vi "TP_Calibration.vi"(9 "PEU":refnum<class "PEU.lvclass">, 10 "TP":string, 11 "E5071C":refnum<class "E5071C.lvclass">) -> (3 "Calibration Done":bool)   [LabVIEW 2020]
uses:
  Driver/E5071C/E5071C/E5071C.lvclass
  Driver/PEU/PEU/PEU.lvclass
panel:
  in  "返回":bool
  in  "THROUGH":bool
  in  "LOAD 2":bool
  in  "SHORT 2":bool
  in  "LOAD 1":bool
  in  "SHORT 1":bool
  in  "OPEN 2":bool
  out "TP1":string
  out "TP2":string
  in  "OPEN 1":bool
  in  "确认":bool
  # "E5071C校准"
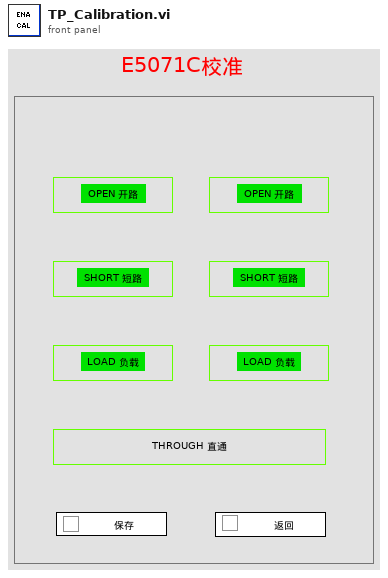
[diagram p1: front panel]
types:
  T1 = enum8{"Enabled", "Disabled", "Disabled and Grayed Out"}
  T2 = cluster{"E5071C":refnum<class "E5071C.lvclass">, "Button Name":string, ":SENS":i32, "Calibration Done":bool, "Done Count":string[]}
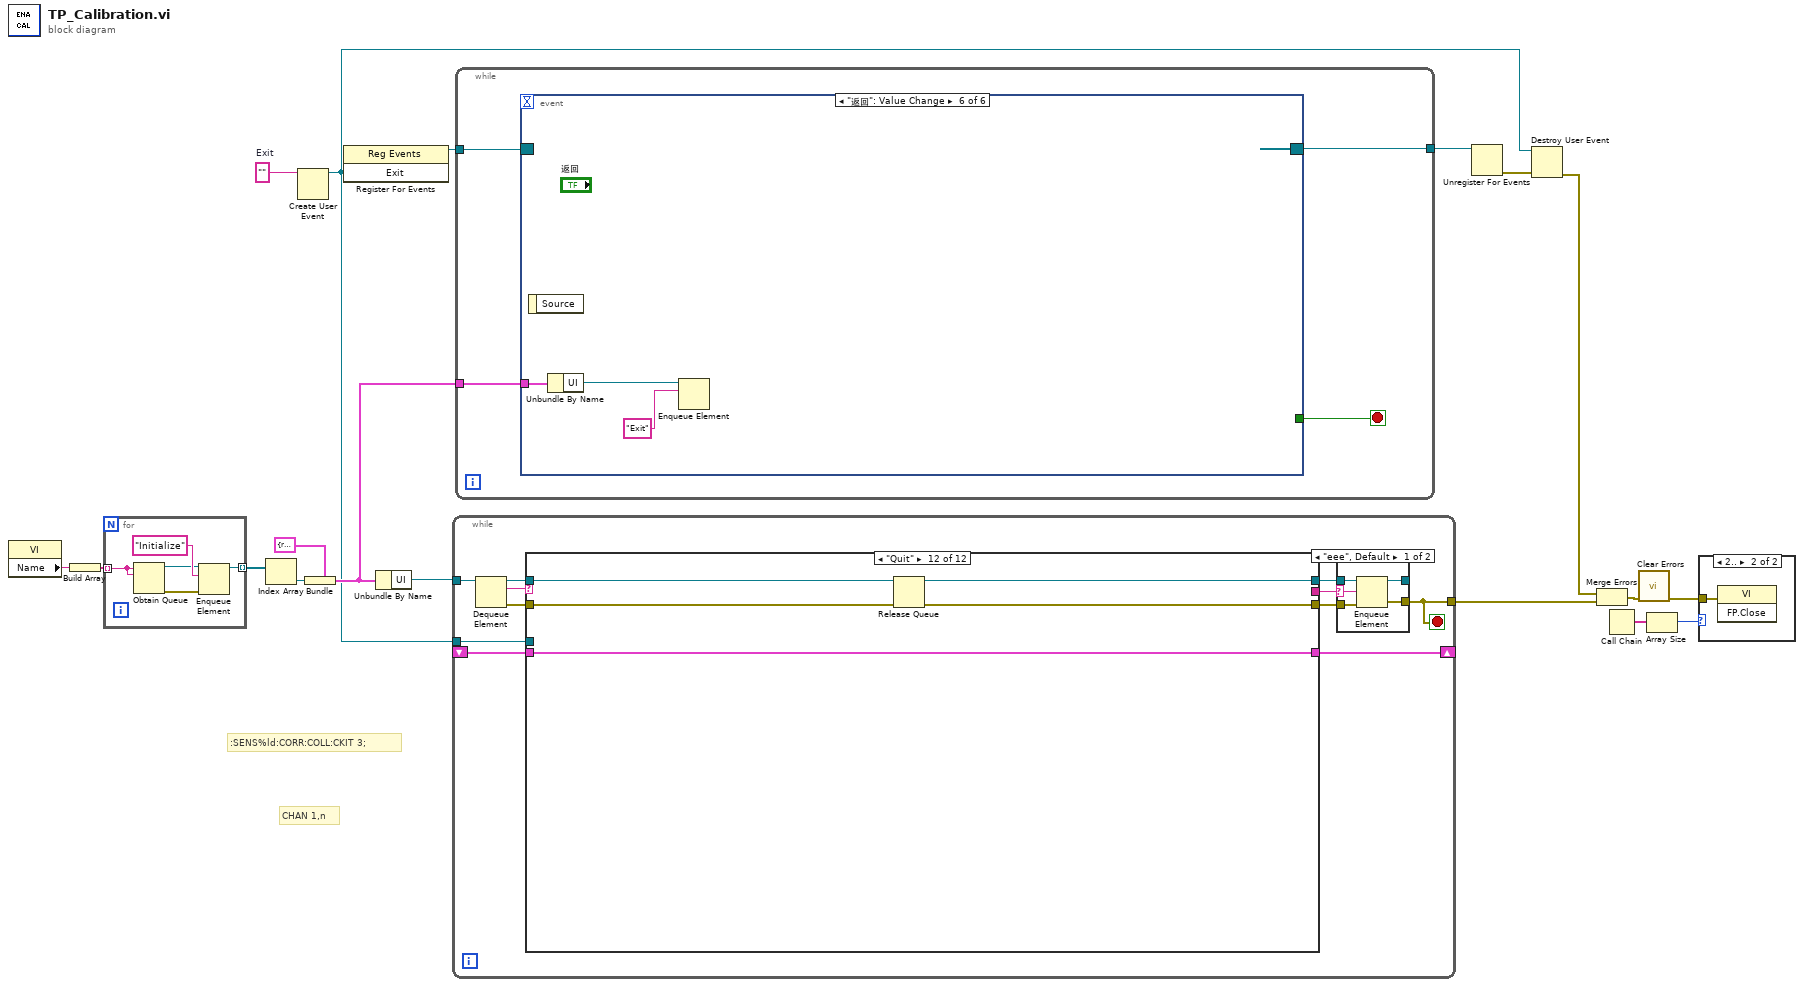
[diagram p0: block diagram]
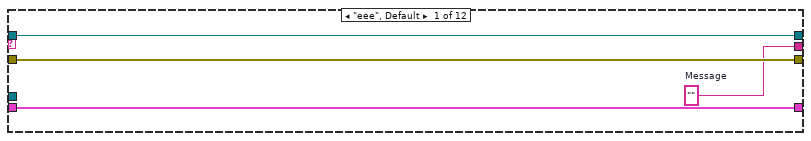
[diagram p4: hidden frame]
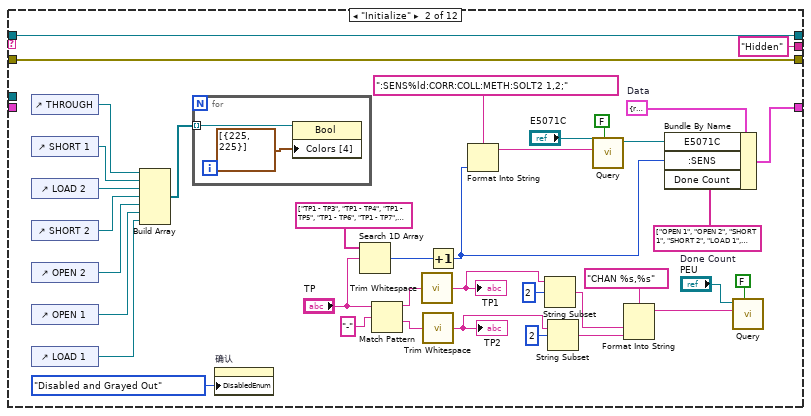
[diagram p5: hidden frame]
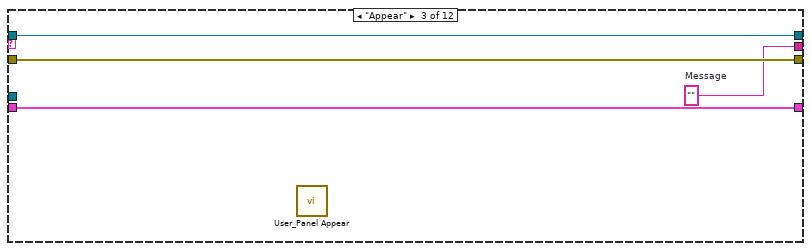
[diagram p6: hidden frame]
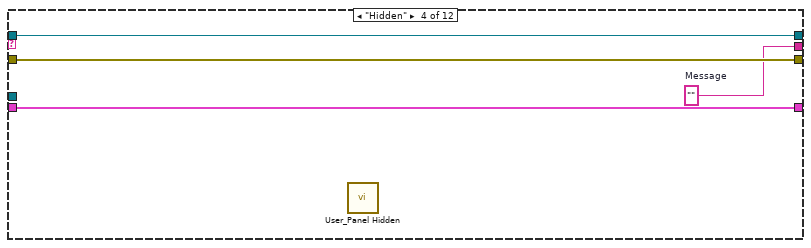
[diagram p7: hidden frame]
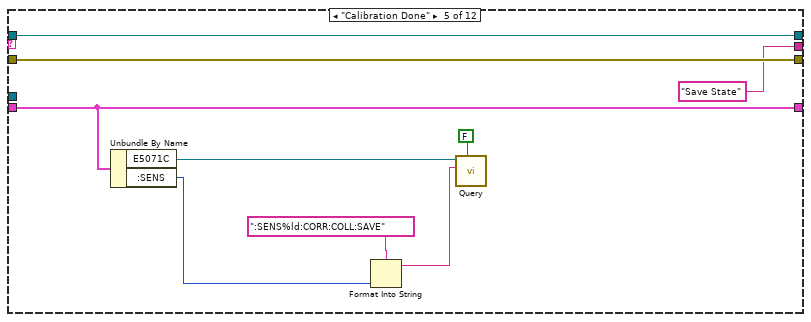
[diagram p8: hidden frame]
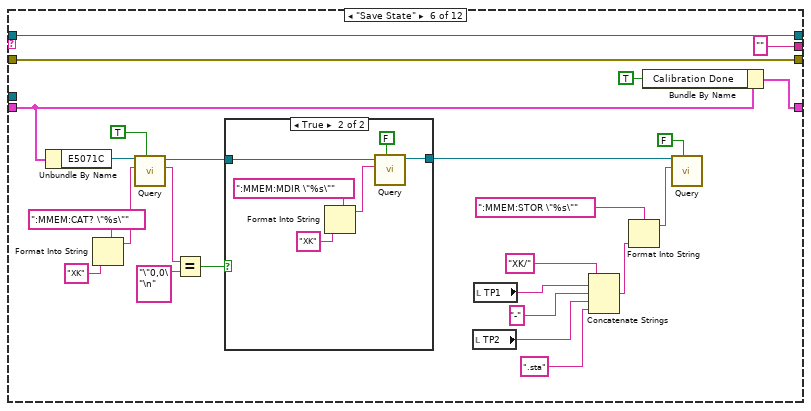
[diagram p9: hidden frame]
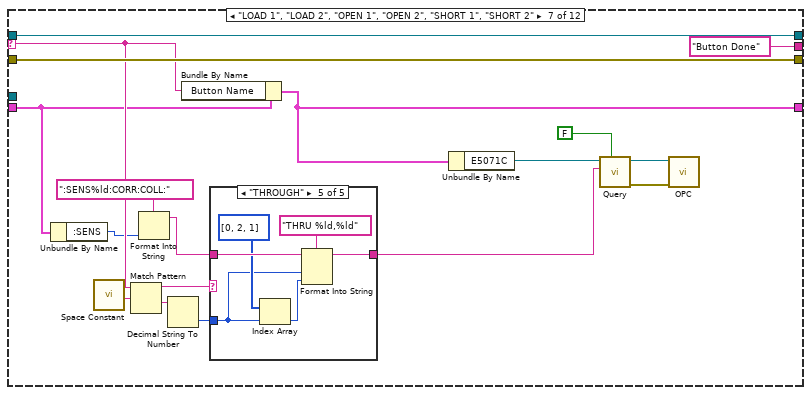
[diagram p11: hidden frame]
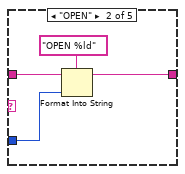
[diagram p13: hidden frame]
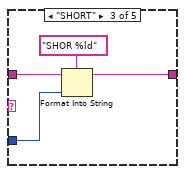
[diagram p14: hidden frame]
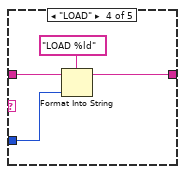
[diagram p15: hidden frame]
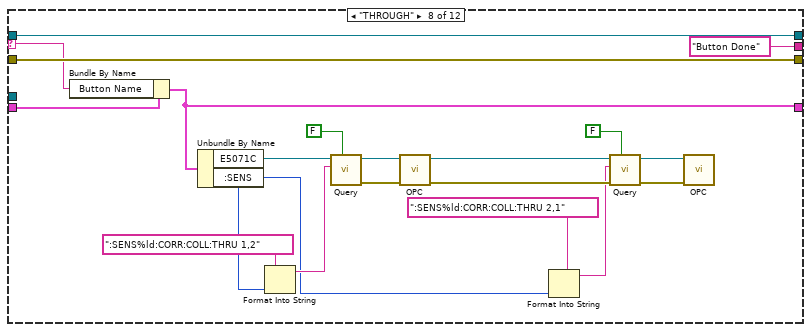
[diagram p16: hidden frame]
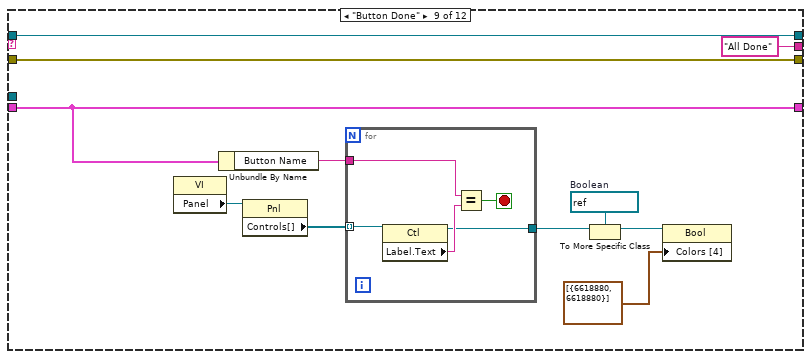
[diagram p17: hidden frame]
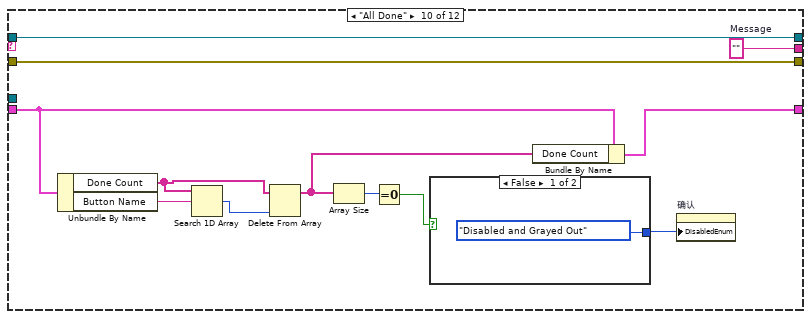
[diagram p18: hidden frame]
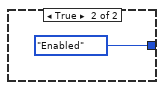
[diagram p19: hidden frame]
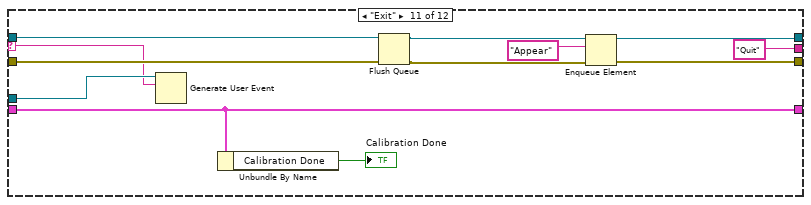
[diagram p20: hidden frame]
diagram:
  w7 = ""  # Exit
  # "CHAN 1,n"
  # ":SENS%ld:CORR:COLL:CKIT 3;"
  n1 = property class="VI"() -> ("Name"=w17:string)  [unwired: 2 in, 2 out]
  n2 = Build Array(w17) -> (w18:string[])
  n3 = for {
    tunnel: w18 -> [w19] mode=indexing
    tunnel: [w20] -> w12 mode=indexing
    n4 = Obtain Queue(name (unnamed)=w19, element data type=w19) -> (queue out=w22:refnum<queue>, error out=w21:errorcluster)  [unwired: 3 in, 1 out]
    n5 = Enqueue Element(queue=w22, element="Initialize" ("元素"), error in (no error)=w21) -> (queue out=w20:refnum<queue>)  [unwired: 1 in, 2 out]
  }
  n6 = Index Array(array=w12) -> (element=w15:refnum<queue>)  [unwired: 1 in]
  n7 = Create User Event(user event datatype=w7) -> (user event=w11:refnum<user-event>)  [unwired: 1 in, 1 out]
  n8 = Bundle(cluster=cluster{"UI":refnum<queue>} {"UI"=refnum}, "UI"=w15) -> (w16:cluster{"UI":refnum<queue>})
  n9 = register-events(w11) -> (reference out=w8:refnum<event-registration>)  [unwired: 2 in, 1 out]
  n10 = Unbundle By Name(w16) -> ("UI"=w13:refnum<queue>)
  n11 = while {
    tunnel: w13 -> [w34]
    tunnel: [w24] -> w1
    shift-right: [w28] -> _
    shift-left: _ -> [w27]
    tunnel: w11 -> [w26]
    stop <- w24 stop-if-true
    n12 = Dequeue Element(queue=w34) -> (queue out=w33:refnum<queue>, element=w25:string, error out=w30:errorcluster)  [unwired: 2 in, 1 out]
    n13 = case shown="\"Quit\"" w25 {
      selector: w25 -> [_ _ _ _ _ _ w142 w184 _ _ w227 _]
      tunnel: w33 -> [w45 w82 w88 w92 w101 w126 w151 w189 w200 w217 w230 w235]
      tunnel: [w45 w82 w88 w92 w101 w126 w151 w189 w200 w217 w222 w235] -> w32
      tunnel: [w44 w81 w87 w91 w100 w125 w150 w188 w199 w216 w224 w232] -> w31
      tunnel: w30 -> [w44 w81 w87 w91 w100 w125 w150 w188 w199 w216 w229 w234]
      tunnel: [w43 "Hidden" ("Message") w86 w90 "Save State" ("Message") "" ("Message") "Button Done" ("Message") "Button Done" ("Message") "All Done" ("Message") w215 "Quit" ("Message") _] -> w29
      tunnel: [w42 w78 w85 w89 w98 w103 w141 w183 w197 w211 w221 w233] -> w28
      tunnel: w27 -> [w42 _ w85 w89 w98 w104 w137 w185 w197 w212 w221 w233]
      tunnel: w26 -> [_ _ _ _ _ _ _ _ _ _ w228 _]
      frame "eee", Default {
        w43 = ""  # Message
      }
      frame "Initialize" {
        w65 = string[] ["OPEN 1", "OPEN 2", "SHORT 1", "SHORT 2", "LOAD 1", "LOAD 2", "THROUGH"]  # Done Count
        w79 = T2 {"E5071C"=refnum, "Button Name"="", ":SENS"=0, "Calibration Done"=FALSE, "Done Count"=["OPEN 1", "OPEN 2", "SHORT 1", "SHORT 2", "LOAD 1", "LOAD 2", "THROUGH"]}  # Data
        n14 = control-ref of="THROUGH"() -> (w63:refnum<vi>)
        n15 = control-ref of="SHORT 1"() -> (w62:refnum<vi>)
        n16 = control-ref of="LOAD 2"() -> (w61:refnum<vi>)
        n17 = control-ref of="SHORT 2"() -> (w60:refnum<vi>)
        n18 = control-ref of="OPEN 2"() -> (w59:refnum<vi>)
        n19 = control-ref of="OPEN 1"() -> (w58:refnum<vi>)
        n20 = control-ref of="LOAD 1"() -> (w57:refnum<vi>)
        n21 = Build Array(w63, w62, w61, w60, w59, w58, w57) -> (w56:refnum<vi>[])
        n22 = for {
          tunnel: w56 -> [w84] mode=indexing
          n23 = property class="Bool"(reference=w84, "Colors [4]"=cluster{u32, u32}[] [{225, 225}]) -> ()  [unwired: 1 in, 2 out]
        }
        n24 = property on="确认" class="Bool"("DisabledEnum"=T1."Disabled and Grayed Out" ("Disabled")) -> ()  [unwired: 2 in, 2 out]
        n25 = Search 1D Array(1D array=string[] ["TP1 - TP3", "TP1 - TP4", "TP1 - TP5", "TP1 - TP6", "TP1 - TP7", "TP1 - TP8", "TP1 - TP9", "TP1 - TP10", "TP1 - TP11", "TP1 - TP12", "TP1 - TP13", "TP1 - TP14", "TP2 - TP3", "TP2 - TP4"], element="TP") -> (index of element=w67:i32)  [unwired: 1 in]
        n26 = Match Pattern(string="TP", regular expression="-") -> (before substring=w76:string, after substring=w75:string)  [unwired: 1 in, 2 out]
        n27 = call <vilib>:"Trim Whitespace.vi"("string"=w76) -> ("trimmed string"=w54:string)  [unwired: 1 in]
        "TP1" <- w54
        n28 = call <vilib>:"Trim Whitespace.vi"("string"=w75) -> ("trimmed string"=w52:string)  [unwired: 1 in]
        "TP2" <- w52
        n29 = Increment(x=w67) -> (x+1=w64:i32)
        n30 = Format Into String(format string=":SENS%ld:CORR:COLL:METH:SOLT2 1,2;", w64) -> (resulting string=w73:string)  [unwired: 2 in, 1 out]
        n31 = String Subset(string=w54, offset (0)=2) -> (substring=w48:string)  [unwired: 1 in]
        n32 = String Subset(string=w52, offset (0)=2) -> (substring=w47:string)  [unwired: 1 in]
        n33 = call "Query.vi"("Return"=FALSE, "Command"=w73, "E5071C in"="E5071C") -> ("E5071C out"=w72:refnum<class "E5071C.lvclass">)  [unwired: 6 in, 2 out]
        n34 = Format Into String(format string="CHAN %s,%s", w48, w47) -> (resulting string=w46:string)  [unwired: 2 in, 1 out]
        n35 = Bundle By Name(cluster=w79, "E5071C"=w72, ":SENS"=w64, "Done Count"=w65) -> (w78:T2)
        n36 = call "Query.vi"("Return"=FALSE, "Command"=w46, "PEU in"="PEU") -> ()  [unwired: 6 in, 3 out]
      }
      frame "Appear" {
        w86 = ""  # Message
        n37 = call "User_Panel Appear.vi"() -> ()  [unwired: 11 in, 1 out]
      }
      frame "Hidden" {
        w90 = ""  # Message
        n38 = call "User_Panel Hidden.vi"() -> ()  [unwired: 11 in, 1 out]
      }
      frame "Calibration Done" {
        n39 = Unbundle By Name(w98) -> ("E5071C"=w97:refnum<class "E5071C.lvclass">, ":SENS"=w94:i32)
        n40 = Format Into String(format string=":SENS%ld:CORR:COLL:SAVE" ("element"), w94) -> (resulting string=w93:string)  [unwired: 2 in, 1 out]
        n41 = call "Query.vi"("Return"=FALSE, "Command"=w93, "E5071C in"=w97) -> ()  [unwired: 6 in, 3 out]
      }
      frame "Save State" {
        n42 = Unbundle By Name(w104) -> ("E5071C"=w122:refnum<class "E5071C.lvclass">)
        n43 = Format Into String(format string=":MMEM:CAT? \"%s\"" ("element"), "XK") -> (resulting string=w117:string)  [unwired: 2 in, 1 out]
        n44 = call "Query.vi"("Return"=TRUE, "Command"=w117, "E5071C in"=w122) -> ("read buffer"=w116:string, "E5071C out"=w121:refnum<class "E5071C.lvclass">)  [unwired: 6 in, 1 out]
        n45 = Equal?(x=w116, y="\"0,0\"\n") -> (x = y?=w105:bool)
        n46 = case shown="True" w105 {
          tunnel: [w127 w129] -> w123
          tunnel: w121 -> [w127 w128]
          frame False {
          }
          frame True {
            n47 = Format Into String(format string=":MMEM:MDIR \"%s\"" ("element"), "XK") -> (resulting string=w131:string)  [unwired: 2 in, 1 out]
            n48 = call "Query.vi"("Return"=FALSE, "Command"=w131, "E5071C in"=w128) -> ("E5071C out"=w129:refnum<class "E5071C.lvclass">)  [unwired: 6 in, 2 out]
          }
        }
        n49 = local read "TP2"() -> (w109:string)
        n50 = local read "TP1"() -> (w111:string)
        n51 = Concatenate Strings("XK/", w111, "-", w109, ".sta") -> (w107:string)
        n52 = Format Into String(format string=":MMEM:STOR \"%s\"" ("element"), w107) -> (resulting string=w106:string)  [unwired: 2 in, 1 out]
        n53 = Bundle By Name(cluster=w104, "Calibration Done"=TRUE) -> (w103:T2)
        n54 = call "Query.vi"("Return"=FALSE, "Command"=w106, "E5071C in"=w123) -> ()  [unwired: 6 in, 3 out]
      }
      frame "LOAD 1", "LOAD 2", "OPEN 1", "OPEN 2", "SHORT 1", "SHORT 2" {
        n55 = Unbundle By Name(w137) -> (":SENS"=w135:i32)
        n56 = call <vilib>:"Space Constant.vi"() -> ("String"=w148:string)
        n57 = Match Pattern(string=w142, regular expression=w148) -> (before substring=w147:string, after substring=w146:string)  [unwired: 1 in, 2 out]
        n58 = Format Into String(format string=":SENS%ld:CORR:COLL:", w135) -> (resulting string=w134:string)  [unwired: 2 in, 1 out]
        n59 = Decimal String To Number(string=w146) -> (number=w145:i32)  [unwired: 2 in, 1 out]
        n60 = Bundle By Name(cluster=w137, "Button Name"=w142) -> (w141:T2)
        n61 = case shown="\"THROUGH\"" w147 {
          tunnel: w145 -> [_ w154 w158 w162 w165]
          tunnel: [_ w153 w157 w161 w168] -> w144
          tunnel: w134 -> [_ w152 w156 w160 w167]
          frame Default {
          }
          frame "OPEN" {
            n62 = Format Into String(format string="OPEN %ld", initial string=w152, w154) -> (resulting string=w153:string)  [unwired: 1 in, 1 out]
          }
          frame "SHORT" {
            n63 = Format Into String(format string="SHOR %ld", initial string=w156, w158) -> (resulting string=w157:string)  [unwired: 1 in, 1 out]
          }
          frame "LOAD" {
            n64 = Format Into String(format string="LOAD %ld", initial string=w160, w162) -> (resulting string=w161:string)  [unwired: 1 in, 1 out]
          }
          frame "THROUGH" {
            n65 = Index Array(array=i32[] [0, 2, 1], index=w165) -> (element=w164:i32)
            n66 = Format Into String(format string="THRU %ld,%ld", initial string=w167, w165, w164) -> (resulting string=w168:string)  [unwired: 1 in, 1 out]
          }
        }
        n67 = Unbundle By Name(w141) -> ("E5071C"=w149:refnum<class "E5071C.lvclass">)
        n68 = call "Query.vi"("Return"=FALSE, "Command"=w144, "E5071C in"=w149) -> ("error out"=w139:errorcluster, "E5071C out"=w138:refnum<class "E5071C.lvclass">)  [unwired: 6 in, 1 out]
        n69 = call "OPC.vi"("error in (no error)"=w139, "E5071C in"=w138) -> ()  [unwired: 8 in, 2 out]
      }
      frame "THROUGH" {
        n70 = Bundle By Name(cluster=w185, "Button Name"=w184) -> (w183:T2)
        n71 = Unbundle By Name(w183) -> ("E5071C"=w187:refnum<class "E5071C.lvclass">, ":SENS"=w170:i32)
        n72 = Format Into String(format string=":SENS%ld:CORR:COLL:THRU 1,2", w170) -> (resulting string=w173:string)  [unwired: 2 in, 1 out]
        n73 = call "Query.vi"("Return"=FALSE, "Command"=w173, "E5071C in"=w187) -> ("error out"=w181:errorcluster, "E5071C out"=w180:refnum<class "E5071C.lvclass">)  [unwired: 6 in, 1 out]
        n74 = call "OPC.vi"("error in (no error)"=w181, "E5071C in"=w180) -> ("error out"=w179:errorcluster, "E5071C out"=w178:refnum<class "E5071C.lvclass">)  [unwired: 8 in]
        n75 = Format Into String(format string=":SENS%ld:CORR:COLL:THRU 2,1", w170) -> (resulting string=w171:string)  [unwired: 2 in, 1 out]
        n76 = call "Query.vi"("Return"=FALSE, "error in (no error)"=w179, "Command"=w171, "E5071C in"=w178) -> ("error out"=w176:errorcluster, "E5071C out"=w175:refnum<class "E5071C.lvclass">)  [unwired: 5 in, 1 out]
        n77 = call "OPC.vi"("error in (no error)"=w176, "E5071C in"=w175) -> ()  [unwired: 8 in, 2 out]
      }
      frame "Button Done" {
        w193 = refnum<vi> refnum  # Boolean
        n78 = property class="VI"() -> ("Panel"=w196:refnum<vi>)  [unwired: 2 in, 2 out]
        n79 = Unbundle By Name(w197) -> ("Button Name"=w195:string)
        n80 = property class="Pnl"(reference=w196) -> ("Controls[]"=w191:refnum<vi>[])  [unwired: 1 in, 2 out]
        n81 = for {
          tunnel: w191 -> [w205] mode=indexing
          tunnel: w195 -> [w203]
          tunnel: [w201] -> w194
          stop <- w202 stop-if-true
          n82 = property class="Ctl"(reference=w205) -> (reference out=w201:refnum<vi>, "Label.Text"=w204:string)  [unwired: 1 in, 1 out]
          n83 = Equal?(x=w203, y=w204) -> (x = y?=w202:bool)
        }
        n84 = To More Specific Class(target class=w193, reference=w194) -> (specific class reference=w192:refnum<vi>)  [unwired: 1 in, 1 out]
        n85 = property class="Bool"(reference=w192, "Colors [4]"=cluster{u32, u32}[] [{6618880, 6618880}]) -> ()  [unwired: 1 in, 2 out]
      }
      frame "All Done" {
        w215 = ""  # Message
        n86 = Unbundle By Name(w212) -> ("Done Count"=w210:string[], "Button Name"=w214:string)
        n87 = Search 1D Array(1D array=w210, element=w214) -> (index of element=w209:i32)  [unwired: 1 in]
        n88 = Delete From Array(array=w210, index=w209) -> (array with subset deleted=w207:string[])  [unwired: 1 in, 1 out]
        n89 = Array Size(array=w207) -> (size(s)=w208:i32)
        n90 = Equal To 0?(x=w208) -> (x = 0?=w206:bool)
        n91 = case shown="False" w206 {
          tunnel: [T1."Disabled and Grayed Out" ("Disabled") T1."Enabled" ("Disabled")] -> w213
          frame False {
          }
          frame True {
          }
        }
        n92 = Bundle By Name(cluster=w212, "Done Count"=w207) -> (w211:T2)
        n93 = property on="确认" class="Bool"("DisabledEnum"=w213) -> ()  [unwired: 2 in, 2 out]
      }
      frame "Exit" {
        n94 = Generate User Event(user event=w228, event data cluster=w227) -> ()  [unwired: 2 in, 2 out]
        n95 = Unbundle By Name(w221) -> ("Calibration Done"=→"Calibration Done":bool)
        n96 = Flush Queue(queue=w230, error in (no error)=w229) -> (queue out=w223:refnum<queue>, error out=w225:errorcluster)  [unwired: 1 out]
        n97 = Enqueue Element(queue=w223, element="Appear" ("元素"), error in (no error)=w225) -> (queue out=w222:refnum<queue>, error out=w224:errorcluster)  [unwired: 1 in, 1 out]
      }
      frame "Quit" {
        n98 = Release Queue(queue=w235, error in (no error)=w234) -> (error out=w232:errorcluster)  [unwired: 1 in, 2 out]
      }
    }
    n99 = case shown="\"eee\", Default" w29 {
      selector: w29 -> [w35 _]
      tunnel: w32 -> [w39 w41]
      tunnel: w31 -> [w38 w40]
      tunnel: [w37 w40] -> w24
      tunnel: [w36 w41] -> _
      frame "eee", Default {
        n100 = Enqueue Element(queue=w39, element=w35, error in (no error)=w38) -> (queue out=w36:refnum<queue>, error out=w37:errorcluster)  [unwired: 1 in, 1 out]
      }
      frame "" {
      }
    }
  }
  n101 = while {
    tunnel: w8 -> [w238]
    tunnel: [w237] -> w10
    tunnel: w16 -> [w236]
    stop <- w239 stop-if-true
    n102 = event shown="[5] \"返回\": Value Change" {
      selector: w238 -> [_ _ _ _ _ _]
      dyn-events: [_ _ _ _ _ _] -> w237
      timeout: _ -> [_ _ _ _ _ _]
      tunnel: [_ w241 _ _ _ _] -> w239
      tunnel: w236 -> [_ _ w245 w253 w256 w259]
      event Timeout {
        n103 = event-data() -> ()  [unwired: 1 in, 1 out]
      }
      event User Event {
        n104 = event-data() -> ("Exit"=w242:string)  [unwired: 1 in]
        n105 = Equal?(x=w242, y="Exit") -> (x = y?=w241:bool)
      }
      event Panel Close? {
        n106 = event-data() -> ()  [unwired: 1 in, 1 out]
        n107 = Cluster To Array(cluster=w245) -> (array=w244:refnum<queue>[])
        n108 = for {
          tunnel: w244 -> [w248] mode=indexing
          tunnel: "Exit" ("元素") -> [w247]
          n109 = Enqueue Element(queue=w248, element=w247) -> ()  [unwired: 2 in, 3 out]
        }
        n110 = event-data("Discard?"=TRUE ("放弃？")) -> ()  [unwired: 1 in, 1 out]
      }
      event "OPEN 1", "OPEN 2", "SHORT 1", "SHORT 2", "LOAD 1", "LOAD 2", "THROUGH": Value Change {
        n111 = event-data() -> ("CtlRef"=w252:refnum<vi>)  [unwired: 1 in]
        n112 = Unbundle By Name(w253) -> ("UI"=w254:refnum<queue>)
        n113 = property class="Bool"(reference=w252) -> (reference out=w251:refnum<vi>, "Label.Text"=w249:string)  [unwired: 1 in, 1 out]
        n114 = Enqueue Element(queue=w254, element=w249) -> ()  [unwired: 2 in, 3 out]
        n115 = property class="Bool"(reference=w251, "Colors [4]"=cluster{u32, u32}[] [{225, 225}]) -> ()  [unwired: 1 in, 2 out]
      }
      event "确认": Value Change {
        n116 = event-data() -> ()  [unwired: 1 in, 1 out]
        n117 = Unbundle By Name(w256) -> ("UI"=w257:refnum<queue>)
        n118 = Enqueue Element(queue=w257, element="Calibration Done") -> ()  [unwired: 2 in, 3 out]
      }
      event "返回": Value Change {
        n119 = event-data() -> ()  [unwired: 1 in, 1 out]
        n120 = Unbundle By Name(w259) -> ("UI"=w260:refnum<queue>)
        n121 = Enqueue Element(queue=w260, element="Exit") -> ()  [unwired: 2 in, 3 out]
      }
    }
  }
  n122 = Unregister For Events(event registration refnum=w10) -> (error out=w9:errorcluster)  [unwired: 1 in]
  n123 = Destroy User Event(user event=w11, error in=w9) -> (error out=w2:errorcluster)
  n124 = Merge Errors(w2, w1) -> (w6:errorcluster)
  n125 = Call Chain() -> (call chain=w4:string[])
  n126 = call <vilib>:"Clear Errors.vi"("error in (no error)"=w6) -> ("error out"=w5:errorcluster)  [unwired: 5 in, 1 out]
  n127 = Array Size(array=w4) -> (size(s)=w3:i32)
  n128 = case shown="2.." w3 {
    tunnel: w5 -> [_ w261]
    frame 0, Default {
    }
    frame 2.. {
      n129 = invoke class="VI" method="FP.Close"(error in=w261) -> ()  [unwired: 2 in, 3 out]
    }
  }
